vi "Conversion of arrays to VArrays.vi"(8 "error in (no error)":errorcluster, 11 "JSON Variant":variant) -> (0 "error out":errorcluster, 3 "VArray to \nbe inserted":variant)   [LabVIEW 2015]
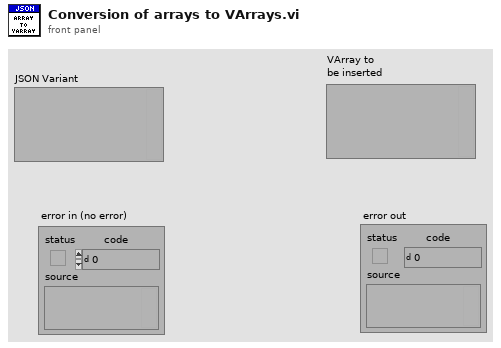
[diagram p1: front panel]
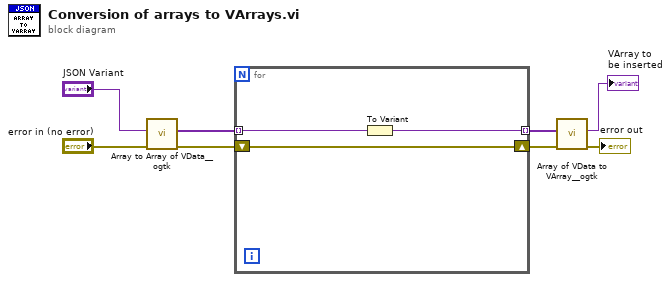
[diagram p0: block diagram]
diagram:
  n1 = call <userlib>:"Array to Array of VData__ogtk.vi"("error in (no error)"="error in (no error)", "MultiD Array"="JSON Variant") -> ("error out"=w6:errorcluster, "1D Array of Variants"=w5:variant[])  [unwired: 8 in]
  n2 = for {
    tunnel: w5 -> [w11] mode=indexing
    tunnel: [w10] -> w3 mode=indexing
    shift-right: [w9] -> w4
    shift-left: w6 -> [w9]
    n3 = To Variant(anything=w11) -> (Variant=w10:variant)
  }
  n4 = call <userlib>:"Array of VData to VArray__ogtk.vi"("error in (no error)"=w4, "1D Array of VData"=w3) -> ("error out"=→"error out":errorcluster, "VArray"=→"VArray to \nbe inserted":variant)  [unwired: 8 in]
